vi "DCPower_MeasureRecordConfiguration.vi"(7 "Aperture Time":dbl, 8 "error in (no error)":errorcluster, 9 "Measure Record Length":i32, 10 "Active Channel Numbers String":string, 11 "IVI Refnum in":refnum<k15>) -> (0 "error out":errorcluster, 2 "aperture time string":string, 3 "IVI Refnum out":refnum<k15>)   [LabVIEW 2019]
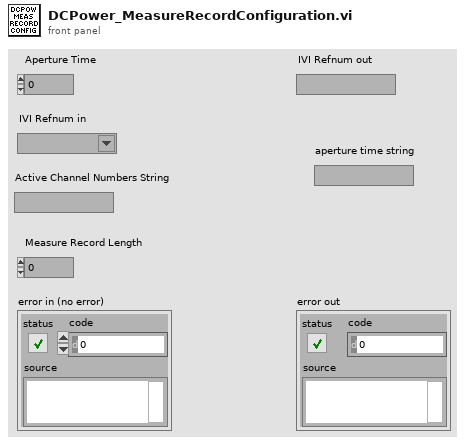
[diagram p1: front panel]
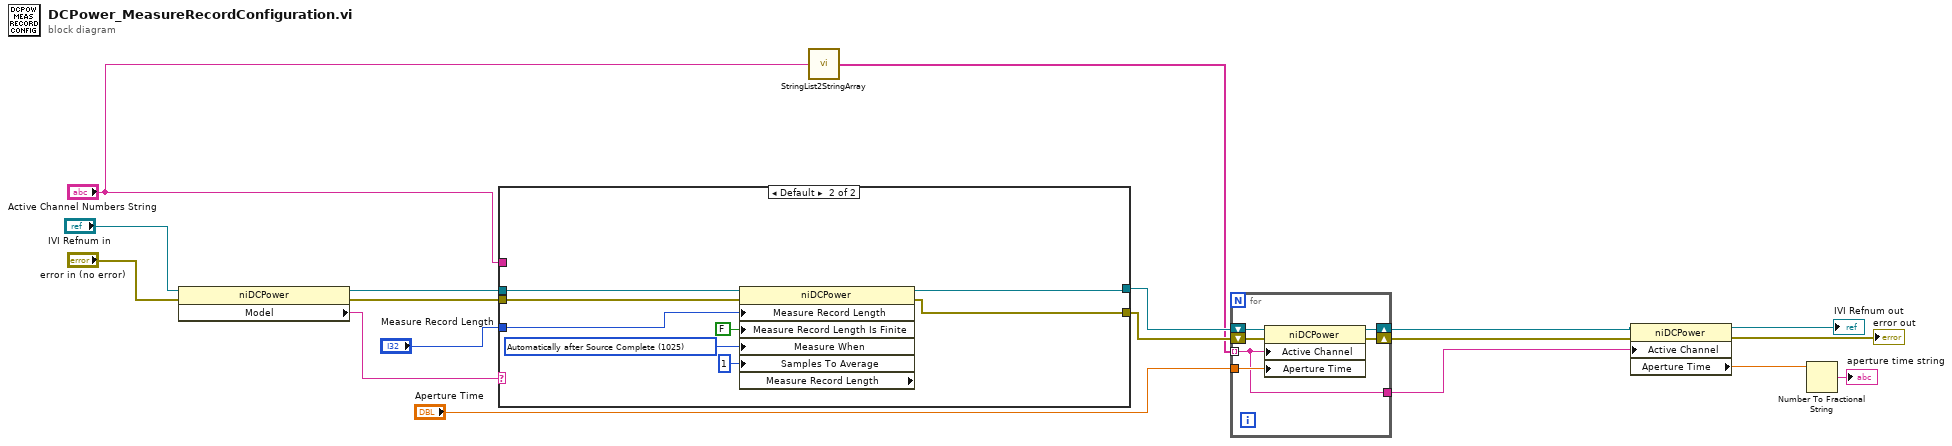
[diagram p0: block diagram]
diagram:
  n1 = property class="niDCPower"(reference="IVI Refnum in", error in="error in (no error)") -> (reference out=w13:refnum<k15>, error out=w14:errorcluster, "Model"=w15:string)
  n2 = case shown="Default" w15 {
    tunnel: [w19 w21] -> w11
    tunnel: [w20 w22] -> w12
    tunnel: "Active Channel Numbers String" -> [_ _]
    tunnel: w13 -> [w20 w25]
    tunnel: w14 -> [w19 w24]
    tunnel: "Measure Record Length" -> [_ w23]
    frame "NI PXI-4110", "NI PXI-4130", "NI PXI-4131A", "NI PXIe-4154" {
    }
    frame Default {
      w27 = 1025 items=["Automatically after Source Complete"=1025, "On Demand"=1026, "On Measure Trigger"=1027] ("Measurement:Advanced:Measure When")
      n3 = property class="niDCPower" props=["Measure Record Length", "Measure Record Length Is Finite", "Measure When", "Samples To Average", "Measure Record Length"](reference=w25, error in=w24, "Measure Record Length"=w23, "Measure Record Length Is Finite"=FALSE ("Measurement:Measure Record Length Is Finite"), "Measure When"=w27, "Samples To Average"=1 ("Measurement:Samples To Average")) -> (reference out=w22:refnum<k15>, error out=w21:errorcluster)  [unwired: 1 out]
    }
  }
  n4 = call "StringList2StringArray.vi"("Active Channel Numbers String"="Active Channel Numbers String") -> ("Array"=w1:string[])
  n5 = for {
    tunnel: "Aperture Time" -> [w32]
    shift-right: [w31] -> w6
    shift-left: w12 -> [w34]
    shift-right: [w30] -> w5
    shift-left: w11 -> [w33]
    tunnel: w1 -> [w29] mode=indexing
    tunnel: [w29] -> w3
    n6 = property class="niDCPower"(reference=w34, error in=w33, "Active Channel"=w29, "Aperture Time"=w32) -> (reference out=w31:refnum<k15>, error out=w30:errorcluster)
  }
  n7 = property class="niDCPower"(reference=w6, error in=w5, "Active Channel"=w3) -> (reference out=→"IVI Refnum out":refnum<k15>, error out=→"error out":errorcluster, "Aperture Time"=w4:dbl)
  n8 = Number To Fractional String(number=w4) -> (F-format string=→"aperture time string":string)  [unwired: 3 in]
